vi "Set Configuration.vi"(8 "error in (no error)":errorcluster, 11 "EST Output in":refnum<class "EST Output.lvclass">) -> (0 "error out":errorcluster, 3 "EST Output out":refnum<class "EST Output.lvclass">)   [LabVIEW 2015, in "EST Output.lvclass"]
uses:
  EST Output.lvclass
  IO Class/Classification.ctl
  Output Signal/Output Signal.lvclass
  IO Class/IO Class.lvclass
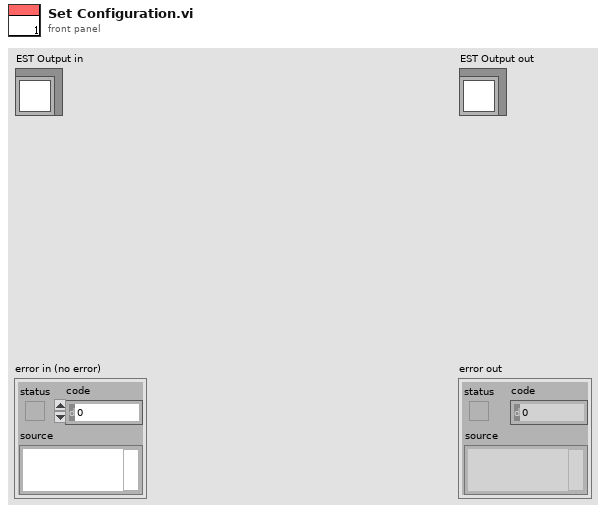
[diagram p1: front panel]
types:
  T1 = typedef "IO Class.lvclass/Classification.ctl" = cluster{"Classification":string}
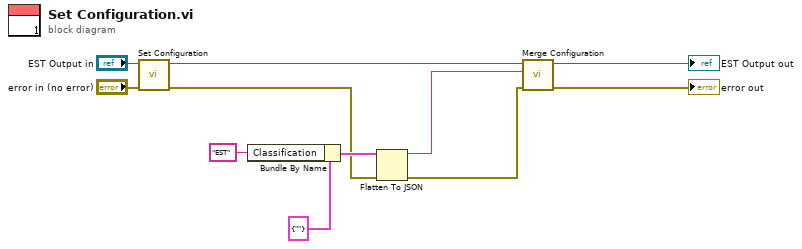
[diagram p0: block diagram]
diagram:
  n1 = call-parent "Set Configuration.vi"("error in (no error)"="error in (no error)", "Output Signal in"="EST Output in") -> ("error out"=w7:errorcluster, "Output Signal out"=w4:refnum<class "EST Output.lvclass">)  [unwired: 8 in]
  n2 = Bundle By Name(cluster=T1 {"Classification"=""} ("Classification"), "Classification"="EST" ("Type")) -> (w8:T1)
  n3 = Flatten To JSON(anything=w8, error in (no error)=w7) -> (JSON string=w2:string, 11:w6:errorcluster)  [unwired: 1 in]
  n4 = call "Merge Configuration.vi"("error in (no error)"=w6, "Additional Configuration"=w2, "IO Class in"=w4) -> ("error out"=→"error out":errorcluster, "IO Class out"=→"EST Output out":refnum<class "EST Output.lvclass">)  [unwired: 7 in]
